vi "Write Timebase.vi"(8 "error in (no error)":errorcluster, 10 "Timebase":T1={"source"="/PXI1Slot6/PXI_Trig1", "rate"=18000000.0}, 11 "NiPxi6733 in":refnum<class "NiPxi6733.lvclass">) -> (0 "error out":errorcluster, 3 "NiPxi6733 out":refnum<class "NiPxi6733.lvclass">)   [LabVIEW 2018, in "FgenPlugins.lvlib" / "NiPxi6733.lvclass"]
uses:
  NiPxi6733.lvclass
  Typedefs/Timebase.ctl
  NiPxi6733.lvclass/NiPxi6733.ctl
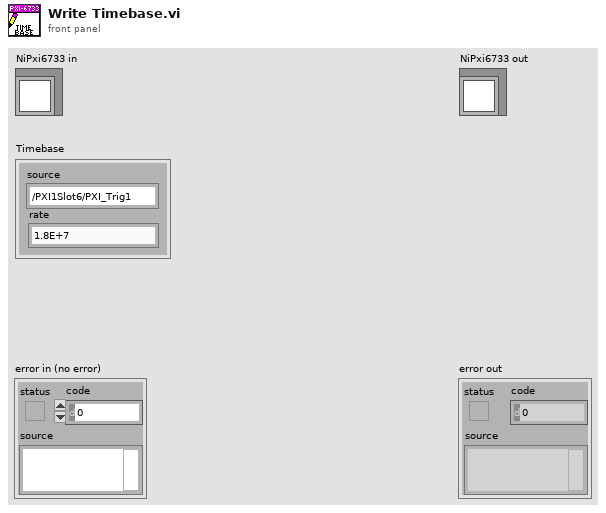
[diagram p1: front panel]
types:
  T1 = typedef "FgenPlugins.lvlib/NiPxi6733.lvclass/Timebase.ctl" = cluster{"source":string, "rate":dbl}
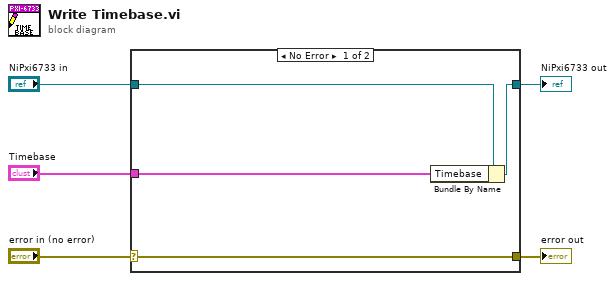
[diagram p0: block diagram]
diagram:
  n1 = case shown="No Error" "error in (no error)" {
    selector: "error in (no error)" -> [w9 w10]
    tunnel: [w9 w10] -> w4
    tunnel: [w7 w11] -> w2
    tunnel: "NiPxi6733 in" -> [w8 w11]
    tunnel: "Timebase" -> [w6 _]
    frame No Error {
      n2 = Bundle By Name(cluster=w8, "Timebase"=w6) -> (w7:refnum<class "NiPxi6733.lvclass">)
    }
    frame Error {
    }
  }
  "error out" <- w4
  "NiPxi6733 out" <- w2
